vi "PMAT_main.vi"() -> ()   [LabVIEW 2019]
uses:
  controls/M1states.ctl
  controls/states.ctl
  controls/holdingRegistersNames.ctl
  <vilib>/NI/Modbus Library/API/Wrapper/Create TCP Master.vi
  <vilib>/ErrorRing/Error Ring.xnode
  <vilib>/NI/Modbus Library/API/Master/Modbus Master.lvclass
  <vilib>/NI/Modbus Library/API/Wrapper/API Main.lvlib
panel:
  out "error IO":errorcluster={"status"=TRUE, "code"=56, "source"="TCP Open Connection in TCP Master.lvclass:Initialize Master.vi->Modbus Master.lvclass:Initialize.vi->API Main.lvlib:Create TCP Master.vi->PMAT_main.vi"}
  out "status":bool
  out "Tab Control":T1(tab)=enum."Page 5"
  out "String 4":string="llenando tanque"
  out "String 2":string="Porfavor introduzca:"
  in  "GRANOS DE MAIZ":bool
  in  "CAL":bool
  out "String":string="BIENVENIDO"
  in  "startCMD":bool
  out "Estado":string
  out "Temperatura":dbl(slide) scale=0.0..100.0
  out "Time":string="00:00"
  out "Multi-Segment Pipe":bool(c317)
  out "Tank 4":dbl(slide) scale=0.0..10.0
  out "Tank 3":dbl(slide) scale=0.0..10.0
  out "filling pot":bool
  out "String 3":string="Por favor espere mientras se configura la máquina"
  in  "close":bool
  out "error out":errorcluster={"status"=TRUE, "code"=5000, "source"="<err>The communication with PLC failed"}
  in  "Stop":bool
  # "°C"
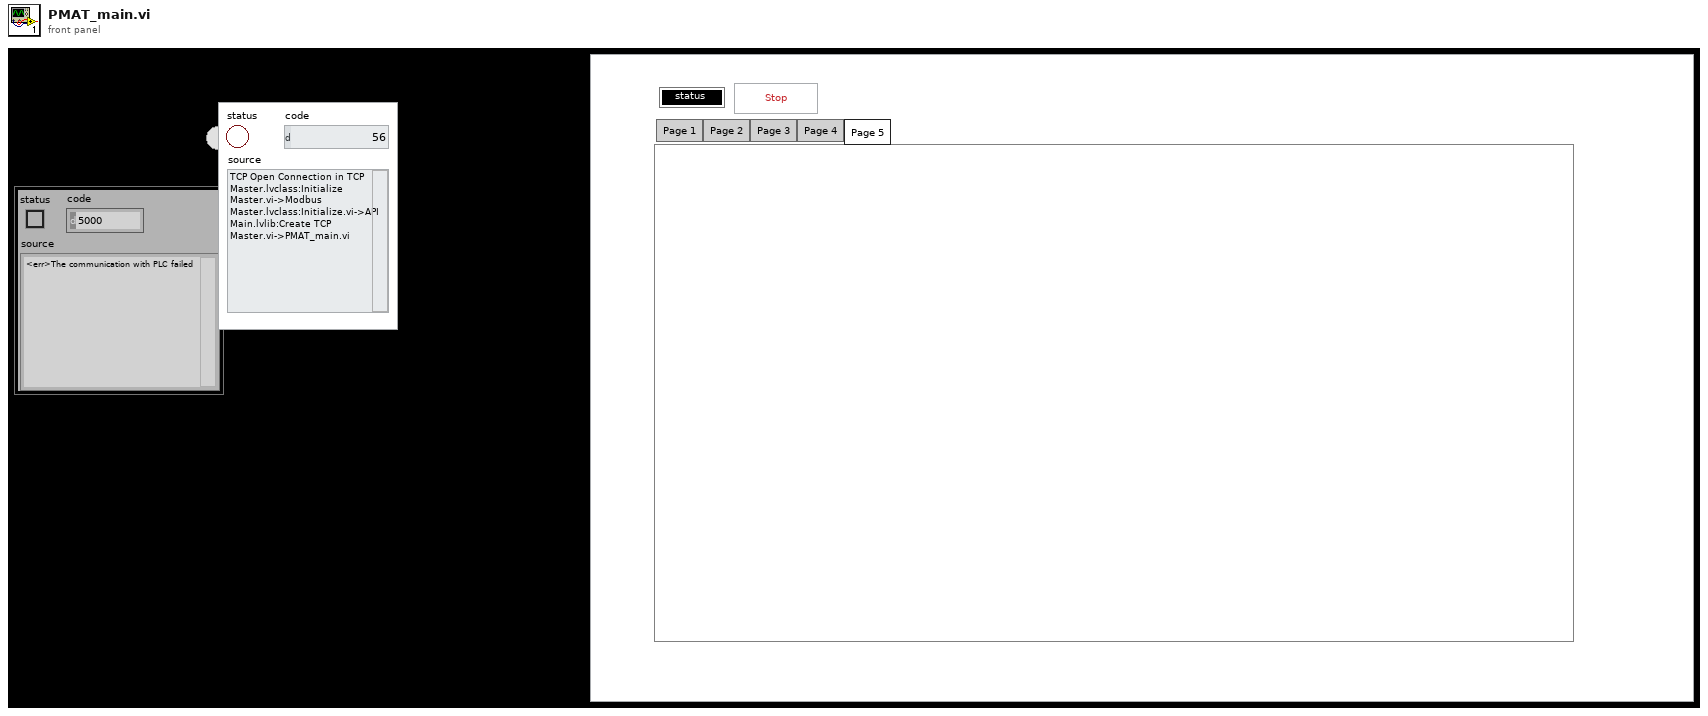
[diagram p1: front panel]
types:
  T1 = enum32{"Page 1", "Page 2", "Page 3", "Page 4", "Page 5"}
  T2 = enum8{"Enabled", "Disabled", "Disabled and Grayed Out"}
  T3 = typedef "states.ctl" = enum16{"Nixtamalización", "Molienda"}
  T4 = typedef "M1states.ctl" = enum16{"VERIFICACION", "PREPARACION", "LAVADO", "CONFIGURANDO"}
  T5 = typedef "holdingRegistersNames.ctl" = u16
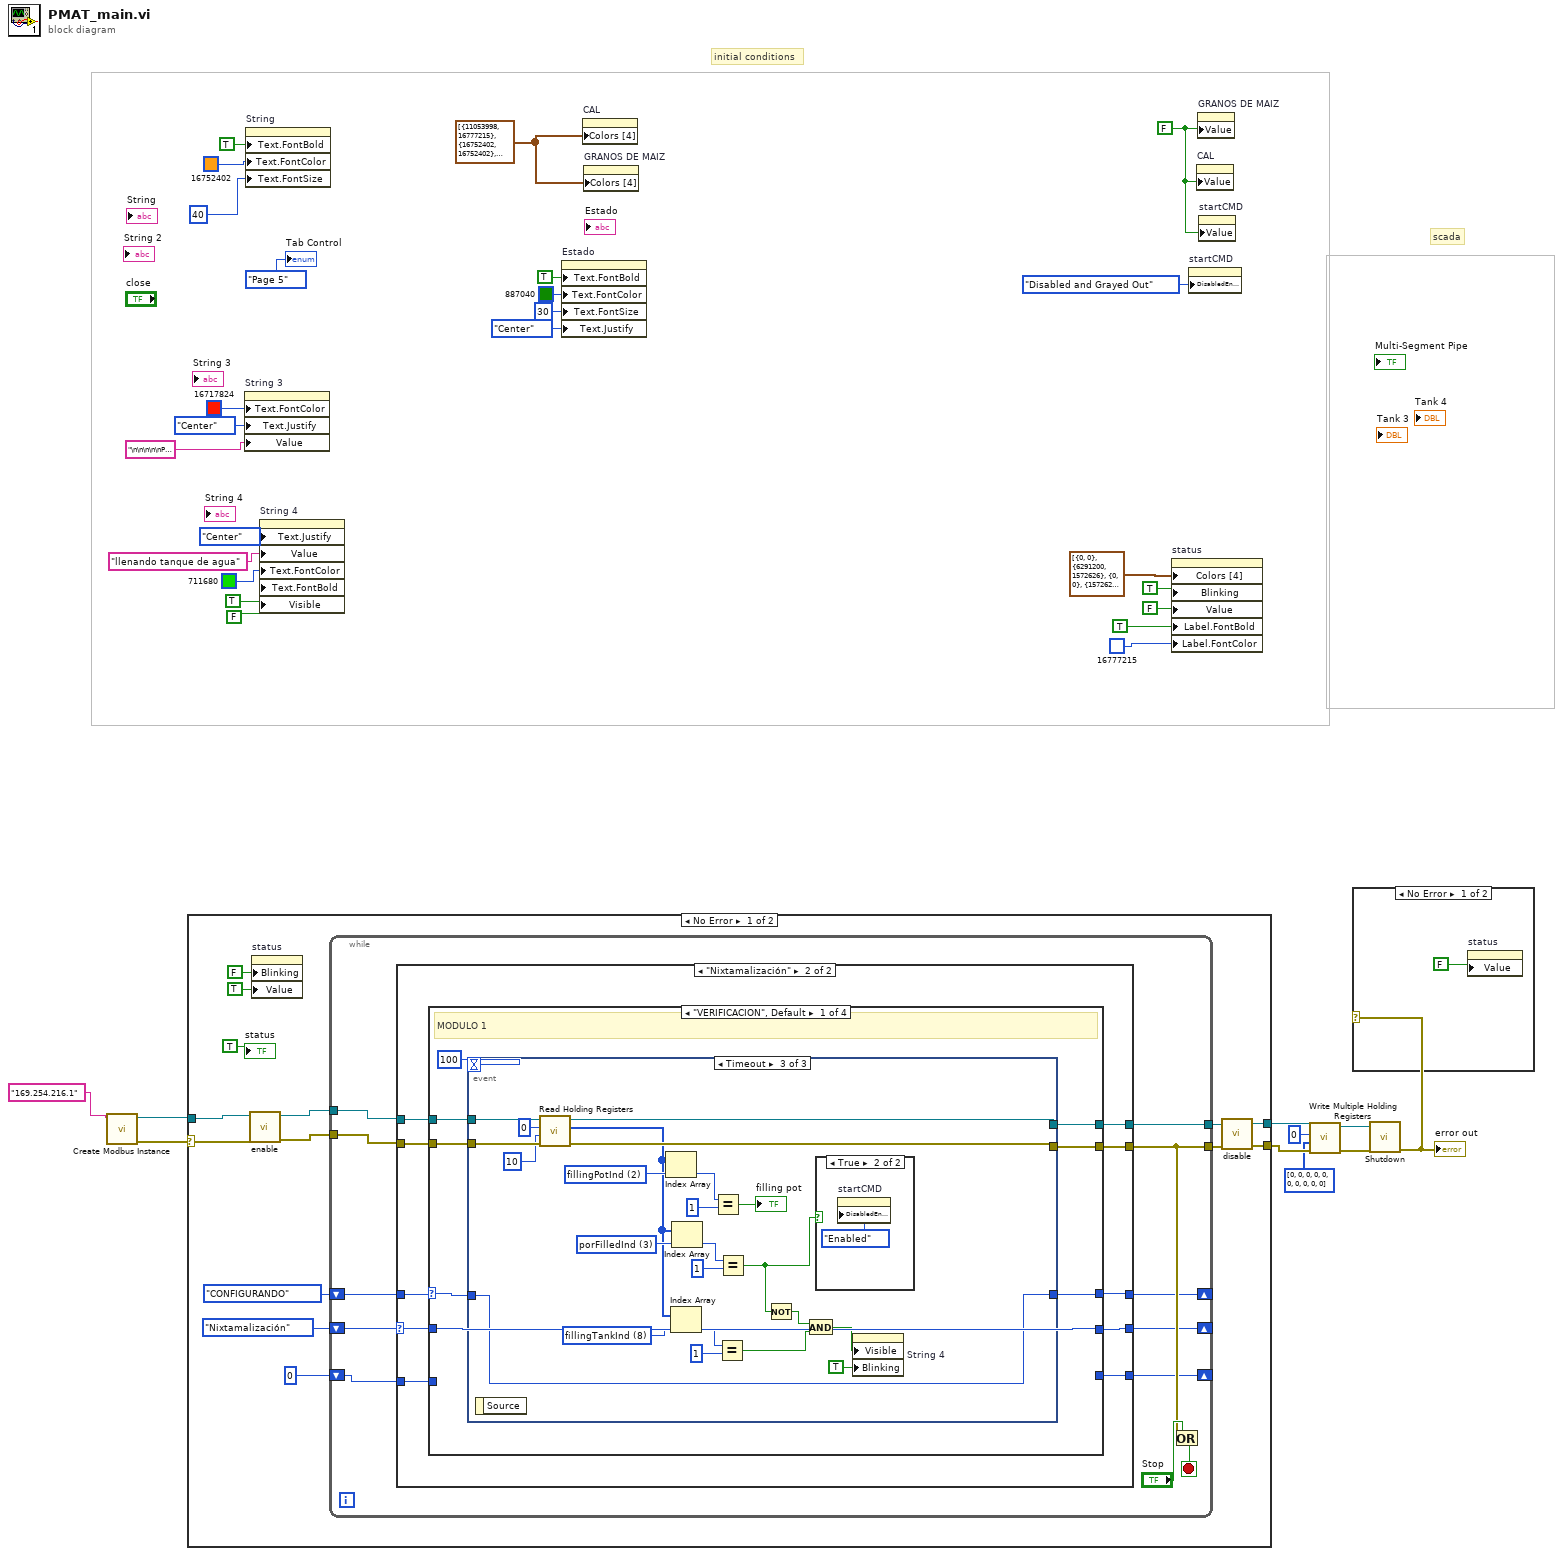
[diagram p0: block diagram]
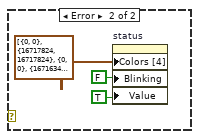
[diagram p2: hidden frame]
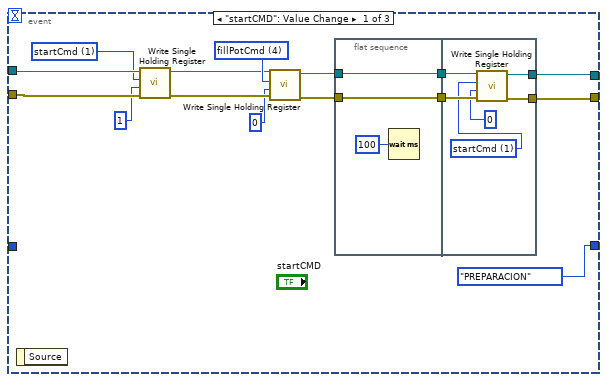
[diagram p4: hidden frame]
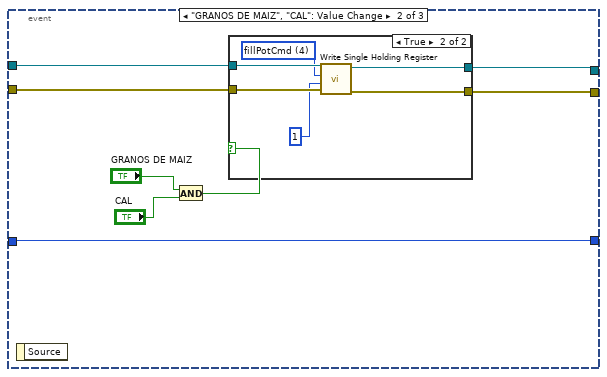
[diagram p5: hidden frame]
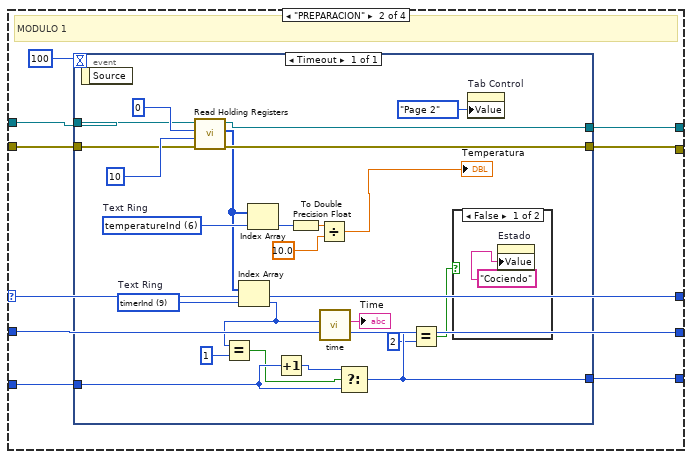
[diagram p8: hidden frame]
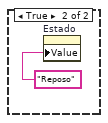
[diagram p9: hidden frame]
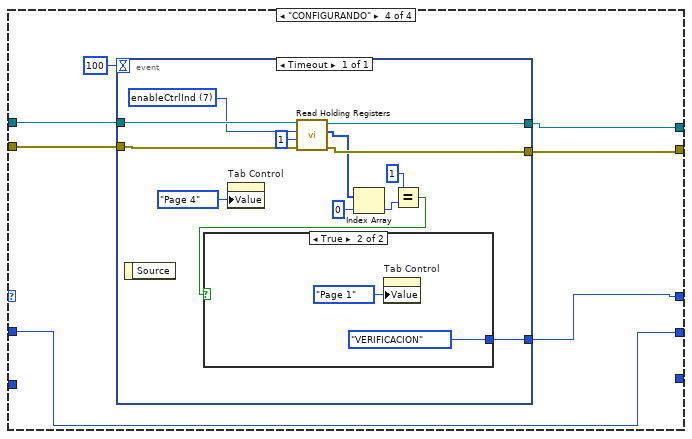
[diagram p11: hidden frame]
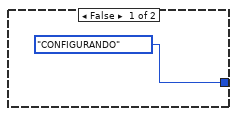
[diagram p12: hidden frame]
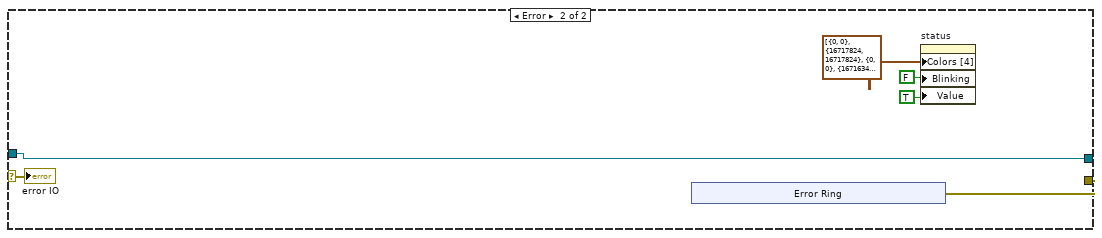
[diagram p13: hidden frame]
diagram:
  w28 = FALSE ("GRANOS DE MAIZ")
  w29 = cluster{"Color Box":u32, "Color Box 2":u32}[] [{"Color Box"=11053998, "Color Box 2"=16777215}, {"Color Box"=16752402, "Color Box 2"=16752402}, {"Color Box"=8224125, "Color Box 2"=16752402}, {"Color Box"=7500402, "Color Box 2"=16448250}, {"Color Box"=0, "Color Box 2"=0}, {"Color Box"=0, "Color Box 2"=0}] ("Colors [4]")
  # "scada"
  # "initial conditions"
  n1 = call-poly <vilib>:"Create Modbus Instance.vi"("address"="169.254.216.1") -> ("error out"=w33:errorcluster, "TCP master instance"=w34:refnum<class "Modbus Master.lvclass">)  [unwired: 9 in]
  n2 = case shown="No Error" w33 {
    selector: w33 -> [w46 w208]
    tunnel: w34 -> [w45 w213]
    tunnel: [w42 w212] -> w8
    tunnel: [w41 w213] -> w9
    frame No Error {
      n3 = call "enable.vi"("Error In"=w46, "Modbus master in"=w45) -> ("Error Out"=w44:errorcluster, "Modbus master out"=w43:refnum<class "Modbus Master.lvclass">)  [unwired: 7 in]
      n4 = property on="status" class="Bool (strict)"("Blinking"=FALSE, "Value"=TRUE ("status")) -> ()  [unwired: 2 in, 2 out]
      n5 = while {
        tunnel: [w58] -> w40
        tunnel: [w57] -> w39
        shift-right: [w54] -> _
        shift-left: M1states."CONFIGURANDO" -> [w56]
        shift-right: [w53] -> _
        shift-left: states."Nixtamalización" -> [w55]
        tunnel: w44 -> [w52]
        tunnel: w43 -> [w51]
        shift-right: [w49] -> _
        shift-left: 0 -> [w50]
        stop <- w59 stop-if-true
        n6 = case shown="\"Nixtamalización\"" w55 {
          selector: w55 -> [w61 w68]
          tunnel: [w64 w74] -> w58
          tunnel: [w63 w73] -> w57
          tunnel: w56 -> [w62 w72]
          tunnel: w51 -> [w64 w71]
          tunnel: w52 -> [w63 w70]
          tunnel: [w62 w67] -> w54
          tunnel: [w61 w69] -> w53
          tunnel: w50 -> [_ w66]
          tunnel: [_ w65] -> w49
          frame "Molienda" {
          }
          frame "Nixtamalización" {
            n7 = case shown="\"VERIFICACION\", Default" w72 {
              selector: w72 -> [w76 w149 w182 _]
              tunnel: w70 -> [w78 w153 w183 w189]
              tunnel: w71 -> [w79 w154 w184 w191]
              tunnel: [w82 w155 w184 w190] -> w74
              tunnel: [w81 w152 w183 w188] -> w73
              tunnel: [w77 w150 w181 w185] -> w69
              tunnel: w68 -> [w77 w150 w181 w185]
              tunnel: [w75 w149 w182 w186] -> w67
              tunnel: w66 -> [_ w148 _ _]
              tunnel: [_ w147 _ _] -> w65
              frame "VERIFICACION", Default {
                # "MODULO 1"
                n8 = event shown="[2] Timeout" {
                  selector: _ -> [_ _ _]
                  dyn-events: _ -> [_ _ _]
                  timeout: 100 -> [_ _ _]
                  tunnel: [w84 w112 w142] -> w82
                  tunnel: [w85 w111 w144] -> w81
                  tunnel: w79 -> [w96 w113 w143]
                  tunnel: w78 -> [w97 w114 w145]
                  tunnel: w76 -> [_ w107 w132]
                  tunnel: [M1states."PREPARACION" w107 w132] -> w75
                  event "startCMD": Value Change {
                    w91 = T5 1 items=["gnrl", "startCmd", "fillingPotInd", "porFilledInd", "fillPotCmd", "TankDrainCmd", ""] ("Text Ring")
                    w94 = T5 4 items=["gnrl", "startCmd", "fillingPotInd", "porFilledInd", "fillPotCmd", "TankDrainCmd", ""] ("Text Ring")
                    n9 = event-data() -> ()  [unwired: 1 in, 1 out]
                    n10 = call-dynamic "Write Single Holding Register.vi"("error in"=w97, "register to write"=u16 1, "address"=w91, "Modbus master in"=w96) -> ("error out"=w95:errorcluster, "Modbus master out"=w92:refnum<class "Modbus Master.lvclass">)  [unwired: 6 in]
                    n11 = call-dynamic "Write Single Holding Register.vi"("error in"=w95, "register to write"=u16 0, "address"=w94, "Modbus master in"=w92) -> ("error out"=w89:errorcluster, "Modbus master out"=w88:refnum<class "Modbus Master.lvclass">)  [unwired: 6 in]
                    n12 = flat-sequence {
                      tunnel: w89 -> [w99]
                      tunnel: w88 -> [w100]
                      tunnel: [w100] -> w87
                      tunnel: [w99] -> w86
                      tunnel: w87 -> [w104]
                      tunnel: w86 -> [w106]
                      tunnel: [w105] -> w85
                      tunnel: [w103] -> w84
                      frame #0 {
                        n13 = Wait (ms)(milliseconds to wait=u32 100) -> ()  [unwired: 1 out]
                      }
                      frame #1 {
                        w102 = T5 1 items=["gnrl", "startCmd", "fillingPotInd", "porFilledInd", "fillPotCmd", "TankDrainCmd", ""] ("Text Ring")
                        n14 = call-dynamic "Write Single Holding Register.vi"("error in"=w106, "register to write"=u16 0, "address"=w102, "Modbus master in"=w104) -> ("error out"=w105:errorcluster, "Modbus master out"=w103:refnum<class "Modbus Master.lvclass">)  [unwired: 6 in]
                      }
                    }
                  }
                  event "GRANOS DE MAIZ", "CAL": Value Change {
                    n15 = event-data() -> ()  [unwired: 1 in, 1 out]
                    n16 = And(x="GRANOS DE MAIZ", y="CAL") -> (x .and. y?=w108:bool)
                    n17 = case shown="True" w108 {
                      tunnel: w114 -> [w115 w122]
                      tunnel: w113 -> [w116 w121]
                      tunnel: [w116 w120] -> w112
                      tunnel: [w115 w119] -> w111
                      frame False {
                      }
                      frame True {
                        w117 = T5 4 items=["gnrl", "startCmd", "fillingPotInd", "porFilledInd", "fillPotCmd", "TankDrainCmd", ""] ("Text Ring")
                        n18 = call-dynamic "Write Single Holding Register.vi"("error in"=w122, "register to write"=u16 1, "address"=w117, "Modbus master in"=w121) -> ("error out"=w119:errorcluster, "Modbus master out"=w120:refnum<class "Modbus Master.lvclass">)  [unwired: 6 in]
                      }
                    }
                  }
                  event Timeout {
                    w128 = T5 8 items=["hmiEnable", "startCmd", "fillingPotInd", "potFilledInd", "fillPotCmd", "TankDrainCmd", "temperatureInd", "enableCtrlInd", "fillingTankInd"] ("Text Ring")
                    w133 = T5 2 items=["gnrl", "startCmd", "fillingPotInd", "porFilledInd", "fillPotCmd", "TankDrainCmd", ""] ("Text Ring")
                    w134 = T5 3 items=["gnrl", "startCmd", "fillingPotInd", "porFilledInd", "fillPotCmd", "TankDrainCmd", ""] ("Text Ring")
                    n19 = event-data() -> ()  [unwired: 1 in, 1 out]
                    n20 = call-dynamic "Read Holding Registers.vi"("error in"=w145, "number of inputs"=u16 10, "starting address"=u16 0, "Modbus master in"=w143) -> ("error out"=w144:errorcluster, "register values"=w129:u16[], "Modbus master out"=w142:refnum<class "Modbus Master.lvclass">)  [unwired: 5 in]
                    n21 = Index Array(array=w129, index=w133) -> (element=w139:u16)
                    n22 = Index Array(array=w129, index=w128) -> (element=w130:u16)
                    n23 = Index Array(array=w129, index=w134) -> (element=w135:u16)
                    n24 = Equal?(x=w139, y=u16 1 ("element")) -> (x = y?=→"filling pot":bool)
                    n25 = Equal?(x=w130, y=u16 1 ("element")) -> (x = y?=w127:bool)
                    n26 = Equal?(x=w135, y=u16 1 ("element")) -> (x = y?=w124:bool)
                    n27 = Not(x=w124) -> (.not. x?=w125:bool)
                    n28 = And(x=w125, y=w127) -> (x .and. y?=w126:bool)
                    n29 = case shown="True" w124 {
                      frame False {
                      }
                      frame True {
                        n30 = property on="startCMD" class="Bool (strict)"("DisabledEnum"=T2."Enabled" ("Disabled")) -> ()  [unwired: 2 in, 2 out]
                      }
                    }
                    n31 = property on="String 4" class="Str"("Visible"=w126, "Blinking"=TRUE) -> ()  [unwired: 2 in, 2 out]
                  }
                }
              }
              frame "PREPARACION" {
                # "MODULO 1"
                n32 = event shown="[0] Timeout" {
                  selector: _ -> [_]
                  dyn-events: _ -> [_]
                  timeout: 100 -> [_]
                  tunnel: [w174] -> w155
                  tunnel: w154 -> [w175]
                  tunnel: w153 -> [w176]
                  tunnel: [w173] -> w152
                  tunnel: w148 -> [w160]
                  tunnel: [w158] -> w147
                  event Timeout {
                    w165 = T5 9 items=["hmiEnable", "startCmd", "fillingPotInd", "potFilledInd", "fillPotCmd", "TankDrainCmd", "temperatureInd", "enableCtrlInd", "fillingTankInd", "timerInd"]  # Text Ring
                    w167 = T5 6 items=["hmiEnable", "startCmd", "fillingPotInd", "potFilledInd", "fillPotCmd", "TankDrainCmd", "temperatureInd", "enableCtrlInd", "fillingTankInd"]  # Text Ring
                    n33 = event-data() -> ()  [unwired: 1 in, 1 out]
                    n34 = call-dynamic "Read Holding Registers.vi"("error in"=w176, "number of inputs"=u16 10, "starting address"=u16 0, "Modbus master in"=w175) -> ("error out"=w173:errorcluster, "register values"=w166:u16[], "Modbus master out"=w174:refnum<class "Modbus Master.lvclass">)  [unwired: 5 in]
                    n35 = Index Array(array=w166, index=w165) -> (element=w163:u16)
                    n36 = Equal?(x=w163, y=u16 1) -> (x = y?=w159:bool)
                    n37 = Index Array(array=w166, index=w167) -> (element=w172:u16)
                    n38 = Increment(x=w160) -> (x+1=w161:i32)
                    n39 = To Double Precision Float(number=w172) -> (double precision float=w171:dbl)
                    n40 = Divide(x=w171, y=10.0) -> (x/y=→"Temperatura":dbl)
                    n41 = call "time.vi"("x"=w163) -> ("Time"=→"Time":string)  [unwired: 10 in]
                    n42 = Select(t=w161, s=w159, f=w160) -> (s? t:f=w158:i32)
                    n43 = Equal?(x=w158, y=2) -> (x = y?=w156:bool)
                    n44 = case shown="False" w156 {
                      frame False {
                        n45 = property on="Estado" class="Str"("Value"="Cociendo" ("Estado")) -> ()  [unwired: 2 in, 2 out]
                      }
                      frame True {
                        n46 = property on="Estado" class="Str"("Value"="Reposo" ("Estado")) -> ()  [unwired: 2 in, 2 out]
                      }
                    }
                    n47 = property on="Tab Control" class="TabCtl (strict)"("Value"=T1."Page 2" ("Tab Control")) -> ()  [unwired: 2 in, 2 out]
                  }
                }
              }
              frame "LAVADO" {
              }
              frame "CONFIGURANDO" {
                n48 = event shown="[0] Timeout" {
                  selector: _ -> [_]
                  dyn-events: _ -> [_]
                  timeout: 100 -> [_]
                  tunnel: [w202] -> w190
                  tunnel: w191 -> [w203]
                  tunnel: w189 -> [w204]
                  tunnel: [w201] -> w188
                  tunnel: [w194] -> w186
                  event Timeout {
                    w193 = T5 7 items=["hmiEnable", "startCmd", "fillingPotInd", "potFilledInd", "fillPotCmd", "TankDrainCmd", "temperatureInd", "enableCtrlInd"] ("Text Ring")
                    n49 = event-data() -> ()  [unwired: 1 in, 1 out]
                    n50 = property on="Tab Control" class="TabCtl (strict)"("Value"=T1."Page 4" ("Tab Control")) -> ()  [unwired: 2 in, 2 out]
                    n51 = call-dynamic "Read Holding Registers.vi"("error in"=w204, "number of inputs"=u16 1, "starting address"=w193, "Modbus master in"=w203) -> ("error out"=w201:errorcluster, "register values"=w199:u16[], "Modbus master out"=w202:refnum<class "Modbus Master.lvclass">)  [unwired: 5 in]
                    n52 = Index Array(array=w199, index=0) -> (element=w197:u16)
                    n53 = Equal?(x=u16 1, y=w197) -> (x = y?=w195:bool)
                    n54 = case shown="True" w195 {
                      tunnel: [M1states."CONFIGURANDO" M1states."VERIFICACION"] -> w194
                      frame False {
                      }
                      frame True {
                        n55 = property on="Tab Control" class="TabCtl (strict)"("Value"=enum32{"Page 1", "Page 2", "Page 3", "Page 4"}."Page 1" ("Tab Control")) -> ()  [unwired: 2 in, 2 out]
                      }
                    }
                  }
                }
              }
            }
          }
        }
        n56 = Or(x=w57, y="Stop") -> (x .or. y?=w59:bool)
      }
      n57 = call "disable.vi"("Error In"=w39, "Modbus master in"=w40) -> ("Error Out"=w42:errorcluster, "Modbus master out"=w41:refnum<class "Modbus Master.lvclass">)  [unwired: 7 in]
      "status" <- TRUE ("Boolean")
    }
    frame Error {
      n58 = xnode "Error Ring"() -> ("error out"=w212:errorcluster)
      n59 = property on="status" class="Bool (strict)"("Colors [4]"=cluster{u32, u32}[] [{0, 0}, {16717824, 16717824}, {0, 0}, {16716346, 16717824}], "Blinking"=FALSE, "Value"=TRUE ("Boolean")) -> ()  [unwired: 2 in, 2 out]
      "error IO" <- w208
    }
  }
  n60 = property on="String 3" class="Str"("Text.FontColor"=u32 16717824, "Text.Justify"=enum16{"Left", "Center", "Right"}."Center" ("Text.Justification"), "Value"="\n\n\n\n\nPor favor espere mientras se configura la máquina" ("String 3")) -> ()  [unwired: 2 in, 2 out]
  n61 = property on="String" class="Str"("Text.FontBold"=TRUE ("Text.Font:Bold"), "Text.FontColor"=u32 16752402, "Text.FontSize"=u32 40 ("Text.Font:Size")) -> ()  [unwired: 2 in, 2 out]
  n62 = property on="String 4" class="Str"("Text.Justify"=enum16{"Left", "Center", "Right"}."Center" ("Text.Justification"), "Value"="llenando tanque de agua" ("String 4"), "Text.FontColor"=u32 711680, "Text.FontBold"=TRUE ("Text.Font:Bold"), "Visible"=FALSE) -> ()  [unwired: 2 in, 2 out]
  n63 = property on="Estado" class="Str"("Text.FontBold"=TRUE ("Text.Font:Bold"), "Text.FontColor"=u32 887040 ("Text.Font:Color"), "Text.FontSize"=u32 30 ("Text.Font:Size"), "Text.Justify"=enum16{"Left", "Center", "Right"}."Center" ("Text.Justification")) -> ()  [unwired: 2 in, 2 out]
  n64 = property on="CAL" class="Bool (strict)"("Colors [4]"=w29) -> ()  [unwired: 2 in, 2 out]
  n65 = property on="GRANOS DE MAIZ" class="Bool (strict)"("Colors [4]"=w29) -> ()  [unwired: 2 in, 2 out]
  n66 = property on="status" class="Bool (strict)"("Colors [4]"=cluster{u32, u32}[] [{0, 0}, {6291200, 1572626}, {0, 0}, {1572626, 1572626}], "Blinking"=TRUE, "Value"=FALSE ("Boolean"), "Label.FontBold"=TRUE ("Label.Font:Bold"), "Label.FontColor"=u32 16777215) -> ()  [unwired: 2 in, 2 out]
  n67 = property on="startCMD" class="Bool (strict)"("DisabledEnum"=T2."Disabled and Grayed Out" ("Disabled")) -> ()  [unwired: 2 in, 2 out]
  n68 = property on="CAL" class="Bool (strict)"("Value"=w28) -> ()  [unwired: 2 in, 2 out]
  n69 = property on="GRANOS DE MAIZ" class="Bool (strict)"("Value"=w28) -> ()  [unwired: 2 in, 2 out]
  n70 = property on="startCMD" class="Bool (strict)"("Value"=w28) -> ()  [unwired: 2 in, 2 out]
  n71 = call-dynamic "Write Multiple Holding Registers.vi"("error in"=w8, "registers to write"=u16[] [0, 0, 0, 0, 0, 0, 0, 0, 0, 0], "starting address"=u16 0, "Modbus master in"=w9) -> ("error out"=w11:errorcluster, "Modbus master out"=w10:refnum<class "Modbus Master.lvclass">)  [unwired: 6 in]
  n72 = call-dynamic "Shutdown.vi"("error in"=w11, "Modbus master in"=w10) -> ("error out"=w5:errorcluster)  [unwired: 9 in]
  "error out" <- w5
  n73 = case shown="No Error" w5 {
    frame No Error {
      n74 = property on="status" class="Bool (strict)"("Value"=FALSE ("Boolean")) -> ()  [unwired: 2 in, 2 out]
    }
    frame Error {
      n75 = property on="status" class="Bool (strict)"("Colors [4]"=cluster{u32, u32}[] [{0, 0}, {16717824, 16717824}, {0, 0}, {16716346, 16717824}], "Blinking"=FALSE, "Value"=TRUE ("Boolean")) -> ()  [unwired: 2 in, 2 out]
    }
  }
  "Tab Control" <- T1."Page 5" ("Tab Control")
